vi "Read Nodes.vi"(8 "error in (no error)":errorcluster, 11 "Messenger Composite in":refnum<class "Messenger Composite.lvclass">) -> (0 "error out":errorcluster, 2 "Nodes":refnum<class "Messenger.lvclass">[](array[class]), 3 "Messenger Composite out":refnum<class "Messenger Composite.lvclass">)   [LabVIEW 2024, in "Messenger Composite.lvclass"]
uses:
  Messenger Composite.lvclass
  Messenger/Messenger.lvclass
  Messenger Composite.lvclass/Messenger Composite.ctl
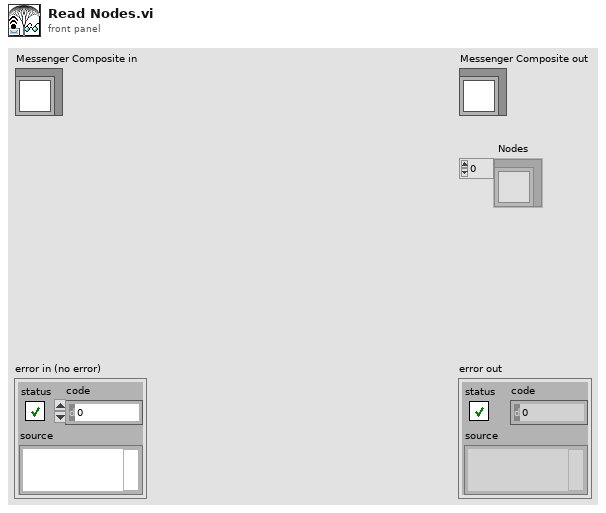
[diagram p1: front panel]
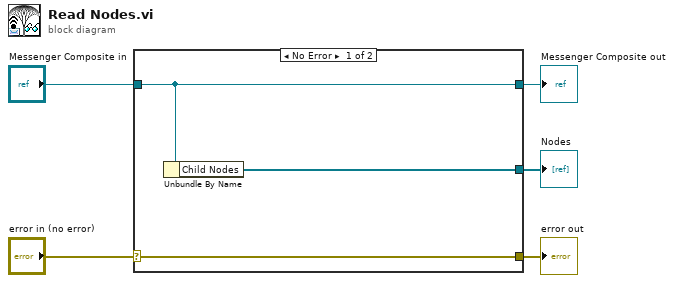
[diagram p0: block diagram]
diagram:
  n1 = case shown="No Error" "error in (no error)" {
    selector: "error in (no error)" -> [w8 w9]
    tunnel: [w8 w9] -> w4
    tunnel: [w7 w10] -> w2
    tunnel: "Messenger Composite in" -> [w7 w10]
    tunnel: [w6 _] -> w1
    frame No Error {
      n2 = Unbundle By Name(w7) -> ("Child Nodes"=w6:refnum<class "Messenger.lvclass">[])
    }
    frame Error {
    }
  }
  "error out" <- w4
  "Messenger Composite out" <- w2
  "Nodes" <- w1
